vi "Rz.vi"(8 "error in (no error)":errorcluster, 9 "Phi":dbl, 10 "Wire in":T1, 11 "Gate in":refnum<class "G-UE.lvclass">) -> (0 "error out":errorcluster, 3 "Gate out":refnum<class "G-UE.lvclass">)   [LabVIEW 2016, in "G-UE.lvclass"]
uses:
  G-UE.lvclass
  TypeDefs/Circuit Cluster.ctl
  GateAbst/GateAbst.lvclass
  <vilib>/Analysis/Matrix/Datatypes/ComplexMatrix.ctl
  <vilib>/Analysis/Matrix/Numeric/Multiply/Multiply - CM,C.vi
  <vilib>/Analysis/Matrix/Numeric/Exponential/Exponential - CM.vi
  <vilib>/Analysis/Matrix/NI_Matrix.lvlib
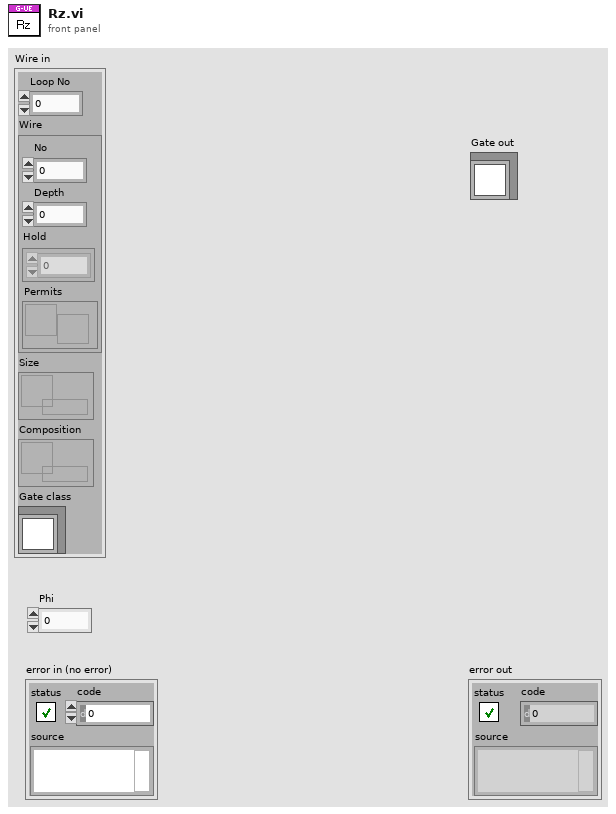
[diagram p1: front panel]
types:
  T1 = typedef "Circuit Cluster.ctl" = cluster{"Loop No":i32, "Wire":cluster{"No":i32, "Depth":i32, "Hold":i32[][], "Permits":refnum<notifier>}, "Size":refnum<queue>, "Composition":refnum<queue>, "Gate class":refnum<class "GateAbst.lvclass">}
  T2 = typedef "NI_Matrix.lvlib/ComplexMatrix.ctl" = cdb[][]
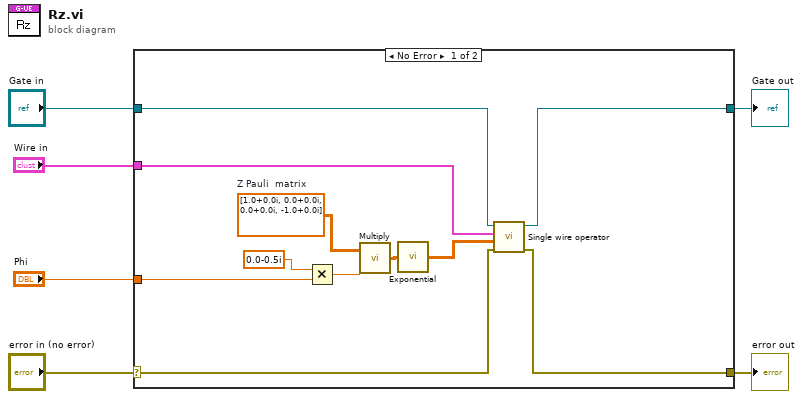
[diagram p0: block diagram]
diagram:
  n1 = case shown="No Error" "error in (no error)" {
    selector: "error in (no error)" -> [w9 w19]
    tunnel: [w10 w19] -> w5
    tunnel: [w11 w18] -> w3
    tunnel: "Gate in" -> [w12 w18]
    tunnel: "Phi" -> [w16 _]
    tunnel: "Wire in" -> [w7 _]
    frame No Error {
      w13 = T2 [[1.0+0.0i, 0.0+0.0i], [0.0+0.0i, -1.0+0.0i]]  # Z Pauli  matrix
      n2 = Multiply ("Multiply.vi")(x=cdb 0.0-0.5i ("Phi"), y=w16) -> (x*y=w14:cdb)
      n3 = call-poly <vilib>:"Multiply.vi"("Complex Scalar c"=w14, "Complex Matrix A"=w13) -> ("A * c"=w15:T2)
      n4 = call-poly <vilib>:"Exponential.vi"("Complex Matrix A"=w15) -> ("e^A"=w8:T2)
      n5 = call "Single wire operator.vi"("error in (no error)"=w9, "Operator matrix"=w8, "Wire in"=w7, "G-UE in"=w12) -> ("error out"=w10:errorcluster, "G-UE out"=w11:refnum<class "G-UE.lvclass">)  [unwired: 6 in]
    }
    frame Error {
    }
  }
  "error out" <- w5
  "Gate out" <- w3
